vi "SetASPIC.vi"(8 "Acquisition Settings":T1, 11 "Aspic Seeting In":T3) -> (0 "error out":errorcluster, 3 "Aspic Seeting Out":T3)   [LabVIEW 2014]
uses:
  AspicSettings.ctl
  AspicMode.ctl
  DAQSettings.ctl
  TriggerMode.ctl
panel:
  out "appended array":u32[](array[numeric])
  out "aspic2Data":u32[](array[numeric])
  out "aspic1Data":u32[](array[numeric])=[8388739, 8454144, 8519680, 3722304989, 4008636142, 4294967295, 10, 10, 10, 10, 10, 10, 10, 10, 10, 10, 10, 10, 10, 10, 10, 10, 10, 10, 10, 10, 10, 10, 10, 10, 10, 10] format="%06x"
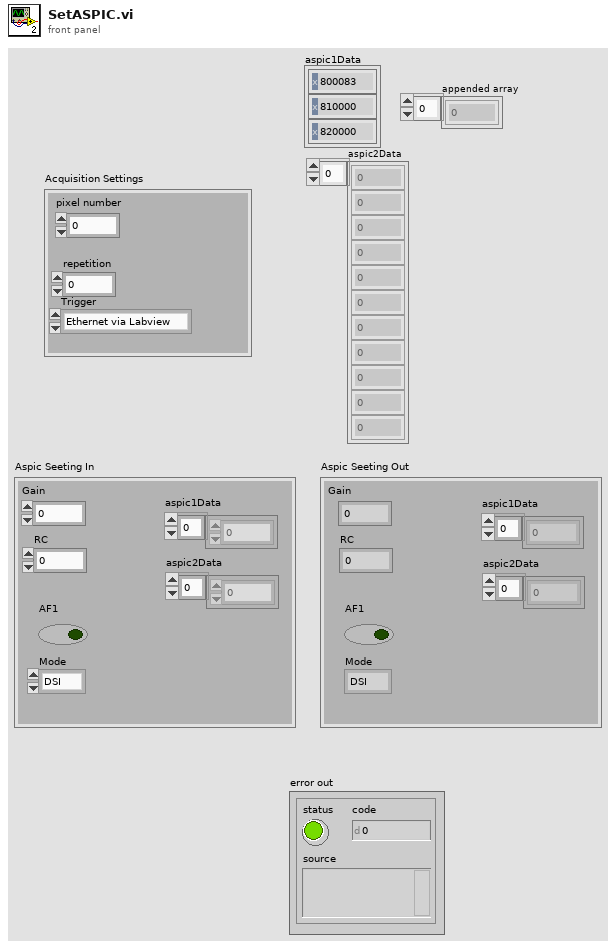
[diagram p1: front panel]
types:
  T1 = typedef "DAQSettings.ctl" = cluster{"pixel number":u32, "repetition":u32, "Trigger":T2}
  T2 = typedef "TriggerMode.ctl" = enum16{"Ethernet via Labview", "SMA (1.8V)"}
  T3 = typedef "AspicSettings.ctl" = cluster{"Gain":u8, "RC":u8, "aspic1Data":u32[], "aspic2Data":u32[], "AF1":bool, "Mode":T4}
  T4 = typedef "AspicMode.ctl" = enum16{"DSI", "TM"}
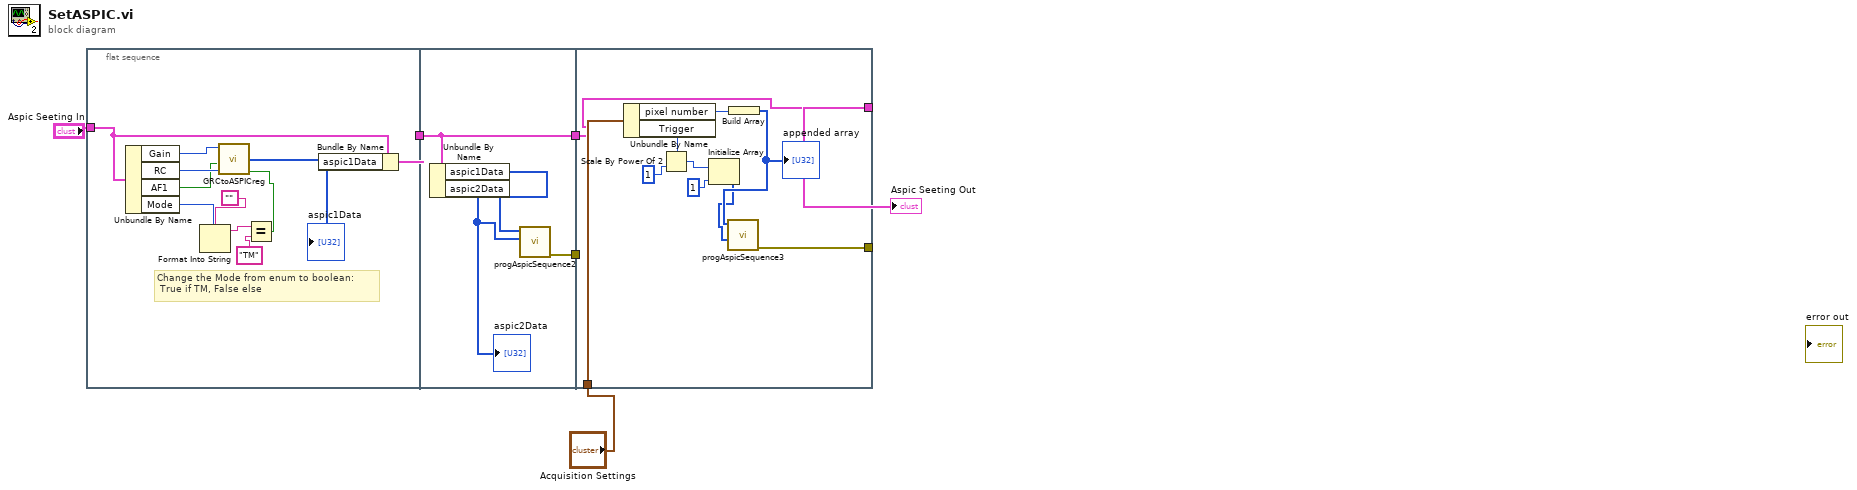
[diagram p0: block diagram]
diagram:
  n1 = flat-sequence {
    tunnel: "Aspic Seeting In" -> [w13]
    tunnel: [w12] -> w5
    tunnel: w5 -> [w21]
    tunnel: [w21] -> w4
    tunnel: [w18] -> w2
    tunnel: w4 -> [w22]
    tunnel: "Acquisition Settings" -> [w31]
    tunnel: w2 -> [_]
    tunnel: [w23] -> _
    tunnel: [w22] -> w1
    frame #0 {
      # "Change the Mode from enum to boolean:\n True if TM, False else"
      n2 = Unbundle By Name(w13) -> ("Gain"=w10:u8, "RC"=w9:u8, "AF1"=w8:bool, "Mode"=w17:T4)
      n3 = Format Into String(format string="", w17) -> (resulting string=w15:string)  [unwired: 2 in, 1 out]
      n4 = Equal?(x=w15, y="TM") -> (x = y?=w7:bool)
      n5 = call "GRCtoASPICreg.vi"("TM"=w7, "AF1"=w8, "RC"=w9, "Gain"=w10) -> ("aspic1Data"=w11:u32[])
      "aspic1Data" <- w11
      n6 = Bundle By Name(cluster=w13, "aspic1Data"=w11) -> (w12:T3)
    }
    frame #1 {
      n7 = Unbundle By Name(w21) -> ("aspic1Data"=w20:u32[], "aspic2Data"=w19:u32[])
      "aspic2Data" <- w19
      n8 = call "progAspicSequence2.vi"("aspic1Data"=w20, "aspic2Data"=w19) -> ("error out"=w18:errorcluster)  [unwired: 7 in]
    }
    frame #2 {
      n9 = Unbundle By Name(w31) -> ("pixel number"=w30:u32, "Trigger"=w29:T2)
      n10 = Scale By Power Of 2(n=w29, x=1) -> (x*2^n=w27:i32)
      n11 = Initialize Array(w27, 1) -> (w24:i32[])
      n12 = Build Array(w30) -> (w25:u32[])
      "appended array" <- w25
      n13 = call "progAspicSequence3.vi"("PixelNumber"=w25, "TriggerSelect"=w24) -> ("error out"=w23:errorcluster)  [unwired: 7 in]
    }
  }
  "Aspic Seeting Out" <- w1
